vi "CtrlTreeAddItemParent.vi"(0 "TreeControl in":refnum<vi>, 1 "Parent Tag":string, 5 "Left Cell String":string, 7 "Child Text":string[](array[string]), 9 "Tag":string, 11 "error in (no error)":errorcluster, 12 "Symbol Index":i32, 13 "Background Color":u32(colorbox)=16777215, 14 "Bold Font":bool) -> (4 "TreeControl out":refnum<vi>, 10 "Tag out":string, 15 "error out":errorcluster)   [LabVIEW 2021]
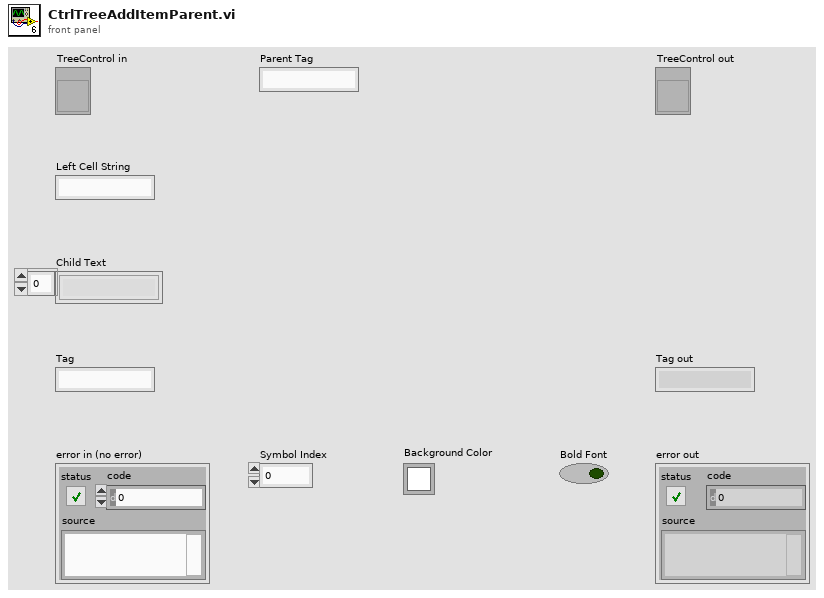
[diagram p1: front panel]
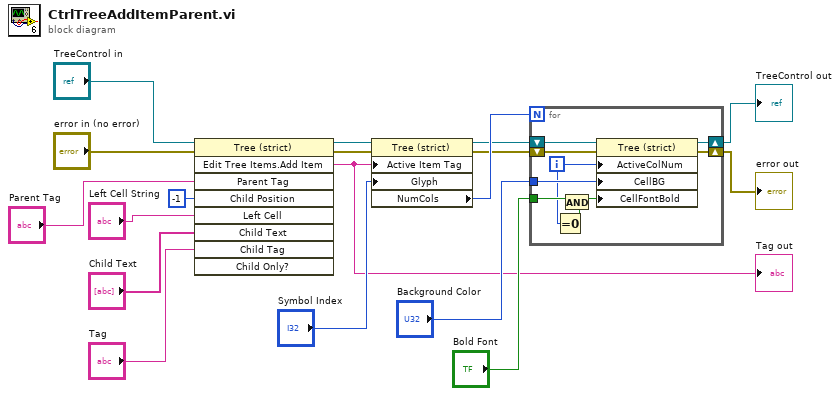
[diagram p0: block diagram]
diagram:
  n1 = invoke class="Tree (strict)" method="Edit Tree Items.Add Item"(reference="TreeControl in", error in="error in (no error)", "Parent Tag"="Parent Tag", "Child Position"=-1, "Left Cell"="Left Cell String", "Child Text"="Child Text", "Child Tag"="Tag") -> (reference out=w8:refnum<vi>, error out=w7:errorcluster, "Edit Tree Items:Add Item"=w3:string)  [unwired: 2 in, 6 out]
  "Tag out" <- w3
  n2 = property class="Tree (strict)"(reference=w8, error in=w7, "Active Item Tag"=w3, "Glyph"="Symbol Index") -> (reference out=w9:refnum<vi>, error out=w10:errorcluster, "NumCols"=w11:u32)
  n3 = for {
    N: w11 -> [_]
    shift-right: [w25] -> w2
    shift-left: w10 -> [w26]
    tunnel: "Background Color" -> [w24]
    shift-right: [w23] -> w1
    shift-left: w9 -> [w27]
    tunnel: "Bold Font" -> [w22]
    i -> [w20]
    n4 = Equal To 0?(x=w20) -> (x = 0?=w19:bool)
    n5 = And(x=w22, y=w19) -> (x .and. y?=w21:bool)
    n6 = property class="Tree (strict)"(reference=w27, error in=w26, "ActiveColNum"=w20, "CellBG"=w24, "CellFontBold"=w21) -> (reference out=w23:refnum<vi>, error out=w25:errorcluster)
  }
  "error out" <- w2
  "TreeControl out" <- w1
